vi "testRemoveIndexOne.vi"(8 "error in (no error)":errorcluster, 11 "TestCase in":refnum<class "ListImp_Populated.lvclass">) -> (0 "error out":errorcluster, 3 "TestCase out":refnum<class "ListImp_Populated.lvclass">)   [LabVIEW 2013, in "ListImp_Populated.lvclass"]
uses:
  ListImp_Populated.lvclass
  ListImp_Populated.lvclass/ListImp_Populated.ctl
  source/LapDog.Collections.Lists/ListImp/ListImp.lvclass
  <vilib>/addons/_JKI Toolkits/VI Tester/TestCase.llb/TestCase.lvclass
  UnitTestComparisons/UnitTestComparisons.lvlib
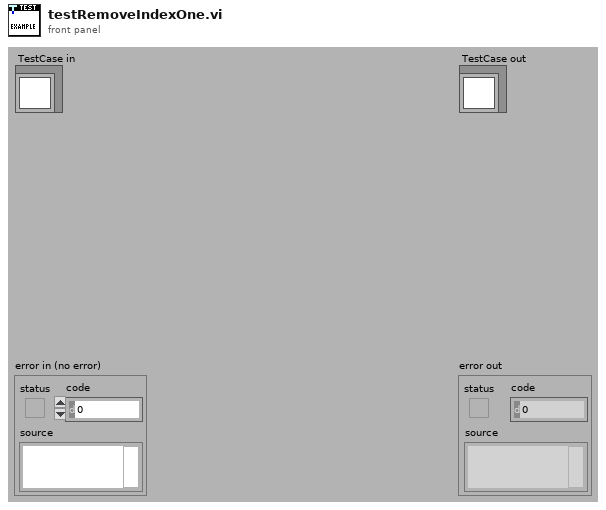
[diagram p1: front panel]
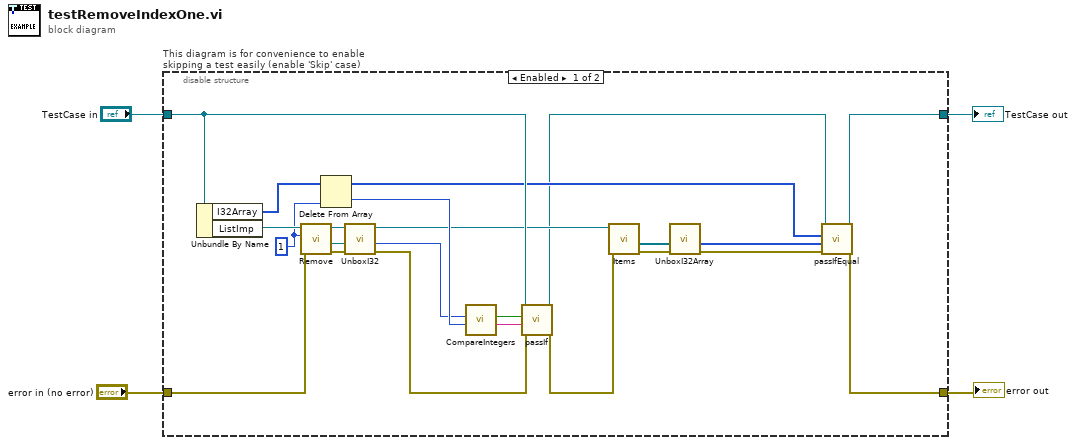
[diagram p0: block diagram]
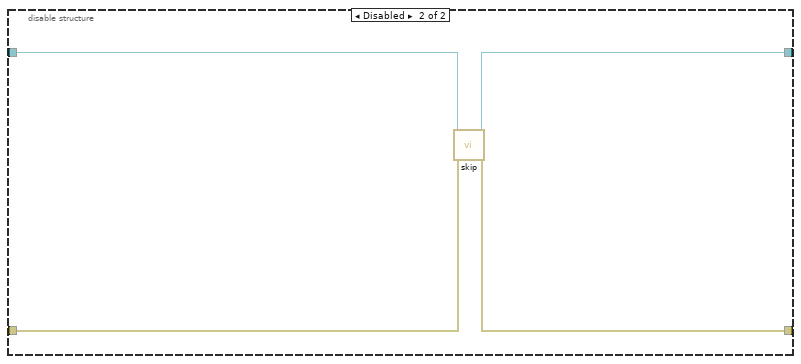
[diagram p2: hidden frame]
diagram:
  n1 = disable-structure "This diagram is for convenience to enable skipping a test easily (enable 'Skip' case)" shown="Enabled" {
    disable-tunnel: "TestCase in" -> [w26 w30]
    disable-tunnel: [w13 w28] -> w1
    disable-tunnel: [w16 w29] -> w3
    disable-tunnel: "error in (no error)" -> [w20 w27]
    frame Enabled {
      w21 = 1 ("Index")
      n2 = Unbundle By Name(w26) -> ("I32Array"=w22:i32[], "ListImp"=w23:refnum<class "ListImp.lvclass">)
      n3 = call-dynamic "Remove.vi"("error in (no error)"=w20, "Index"=w21, "ListImp in"=w23) -> ("error out"=w8:errorcluster, "Item"=w7:refnum<class>, "ListImp out"=w18:refnum<class "ListImp.lvclass">)  [unwired: 6 in]
      n4 = Delete From Array(array=w22, index=w21) -> (deleted portion=w19:i32, array with subset deleted=w15:i32[])  [unwired: 1 in]
      n5 = call "UnboxI32.vi"("error in (no error)"=w8, "Item"=w7) -> ("error out"=w5:errorcluster, "Value"=w6:i32)  [unwired: 8 in]
      n6 = call "CompareIntegers.vi"("Expected Value"=w19, "Actual Value"=w6) -> ("Message"=w24:string, "Equal?"=w25:bool)  [unwired: 8 in]
      n7 = call-dynamic "passIf.vi"("error in (no error)"=w5, "message (\"\")"=w24, "pass"=w25, "TestCase in"=w26) -> ("error out"=w17:errorcluster, "TestCase out"=w14:refnum<class "ListImp_Populated.lvclass">)  [unwired: 6 in]
      n8 = call-dynamic "Items.vi"("error in (no error)"=w17, "ListImp in"=w18) -> ("error out"=w12:errorcluster, "Items"=w11:refnum<class>[])  [unwired: 7 in, 1 out]
      n9 = call "UnboxI32Array.vi"("error in (no error)"=w12, "Items"=w11) -> ("error out"=w10:errorcluster, "Array"=w9:i32[])  [unwired: 8 in]
      n10 = call-dynamic "passIfEqual.vi"("error in (no error)"=w10, "y"=w9, "x"=w15, "TestCase in"=w14) -> ("error out"=w16:errorcluster, "TestCase out"=w13:refnum<class "ListImp_Populated.lvclass">)  [unwired: 6 in]
    }
    frame Disabled {
      # "skip test result while test is under development"
      n11 = call <vilib>:"skip.vi"("error in (no error)"=w27, "TestCase in"=w30) -> ("error out"=w29:errorcluster, "TestCase out"=w28:refnum<class "ListImp_Populated.lvclass">)  [unwired: 8 in]
    }
  }
  "error out" <- w3
  "TestCase out" <- w1
